vi "GetChannelParameters(All).vi"(8 "error in (no error)":errorcluster, 11 "TektronixDPO_PhysicalDevice in":refnum<class "TektronixDPO_PhysicalDevice.lvclass">) -> (0 "error out":errorcluster, 2 "Response":string, 3 "TektronixDPO_PhysicalDevice out":refnum<class "TektronixDPO_PhysicalDevice.lvclass">)   [LabVIEW 2013, in "TektronixDPO_PhysicalDevice.lvclass"]
uses:
  TektronixDPO_PhysicalDevice.lvclass
  TektronixDPO_PhysicalDevice.lvclass/TektronixDPO_PhysicalDevice.ctl
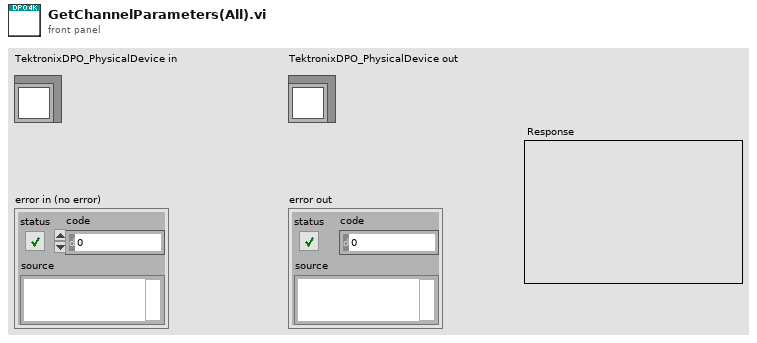
[diagram p1: front panel]
types:
  T1 = typedef "Choice80.ctl" = u16
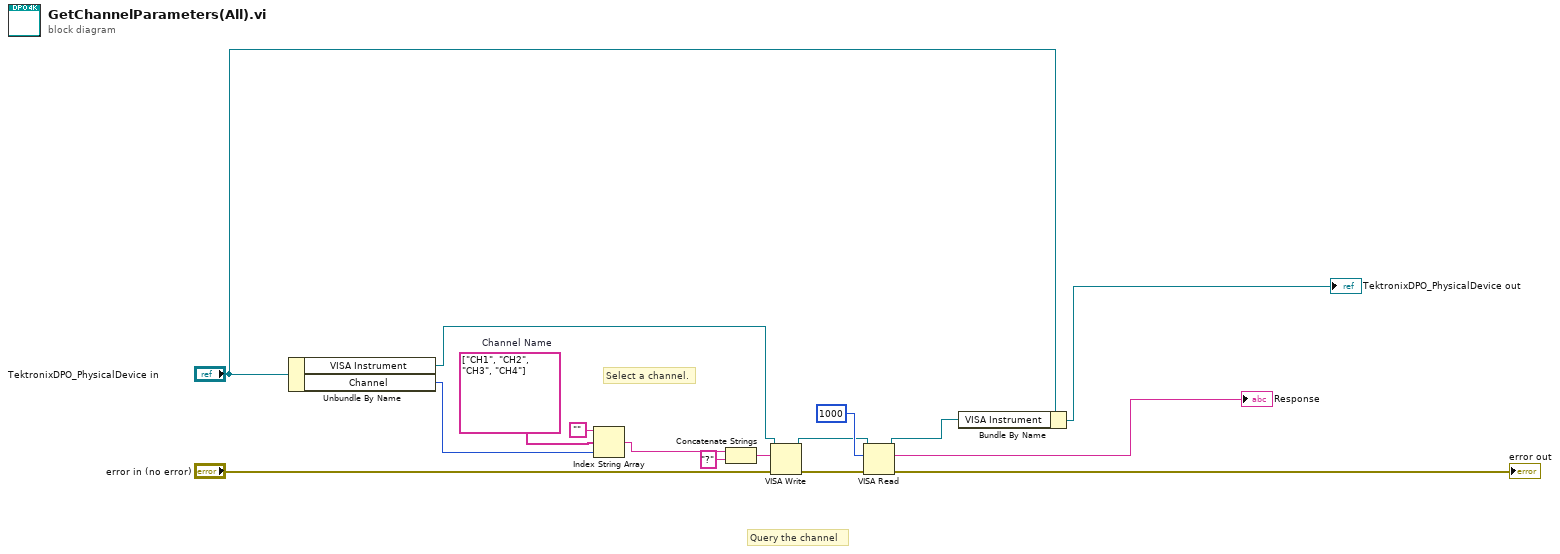
[diagram p0: block diagram]
diagram:
  w8 = string[] ["CH1", "CH2", "CH3", "CH4"]  # Channel Name
  # "Query the channel"
  # "Select a channel."
  n1 = Unbundle By Name("TektronixDPO_PhysicalDevice in") -> ("VISA Instrument"=w12:refnum<visa-resource-name>, "Channel"=w11:T1)
  n2 = Index String Array(1:w11, 2:w8, 3:"") -> (0:w9:string)
  n3 = Concatenate Strings(w9, "?" ("string")) -> (w10:string)
  n4 = VISA Write(VISA resource name=w12, write buffer=w10, error in (no error)="error in (no error)") -> (VISA resource name out=w4:refnum<visa-resource-name>, error out=w6:errorcluster)  [unwired: 1 out]
  n5 = VISA Read(VISA resource name=w4, byte count=u32 1000, error in (no error)=w6) -> (VISA resource name out=w14:refnum<visa-resource-name>, read buffer=→"Response":string, error out=→"error out":errorcluster)  [unwired: 1 out]
  n6 = Bundle By Name(cluster="TektronixDPO_PhysicalDevice in", "VISA Instrument"=w14) -> (→"TektronixDPO_PhysicalDevice out":refnum<class "TektronixDPO_PhysicalDevice.lvclass">)
